vi "Read.vi"(8 "Error In":errorcluster, 10 "Max Data Length":i32=1024, 11 "SFTP File In":refnum<class "SFTP File.lvclass">) -> (0 "Error Out":errorcluster, 2 "Data":u8[](array[numeric]), 3 "SFTP File Out":refnum<class "SFTP File.lvclass">)   [LabVIEW 2021, in "Field_RnD_Services_LIBSSH2_Toolkit.lvlib" / "SFTP File.lvclass"]
doc: "Reads the contents of a remote SFTP file."
uses:
  SFTP File.lvclass
  SFTP File.lvclass/SFTP File.ctl
  Field_RnD_Services_LIBSSH2_Toolkit.lvlib
  SFTP/SFTP.lvclass
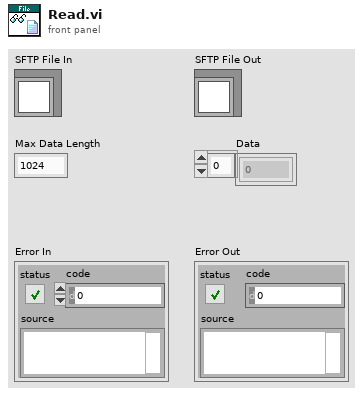
[diagram p1: front panel]
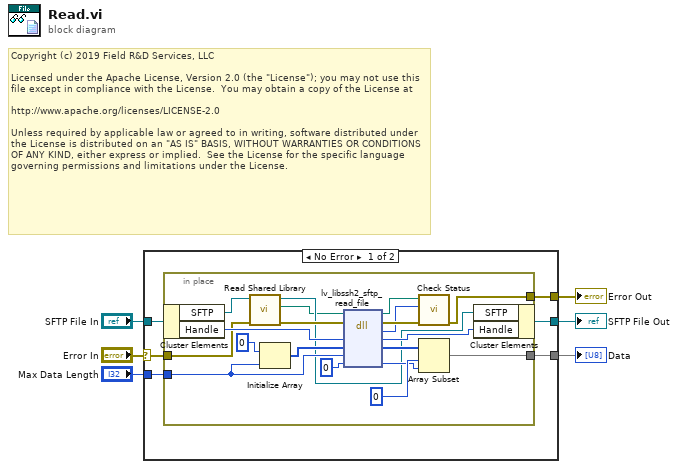
[diagram p0: block diagram]
diagram:
  # "Copyright (c) 2019 Field R&D Services, LLC\n\nLicensed under the Apache License, Version 2.0 (the \"License\"); you may not use this file except in compliance with the License.  You may obtain a copy of the License at\n\nhttp://www.apache.org/licenses/LICENSE-2.0\n\nUnless required by applicable law or agreed to in writing, software distributed under the License is distributed on an \"AS IS\" BASIS, WITHOUT WARRANTIES OR CONDITIONS OF ANY KIND, either express or implied.  See the License for the specific language governing permissions and limitations under the License."
  n1 = case shown="No Error" "Error In" {
    selector: "Error In" -> [w11 w32]
    tunnel: "SFTP File In" -> [w12 w33]
    tunnel: [w10 w33] -> w3
    tunnel: [w7 w32] -> w4
    tunnel: [w9 _] -> w2
    tunnel: "Max Data Length" -> [w8 _]
    frame No Error {
      n2 = in-place {
        in-place-border: w11 -> [w30]
        in-place-border: [w19] -> w9
        in-place-border: w8 -> [w23]
        in-place-border: [w13] -> w7
        n3 = in-place-cluster #1(w12) -> ("SFTP"=w16:refnum<class "SFTP.lvclass">, "Handle"=w31:u64)
        n4 = call "Read Shared Library.vi"("Error In"=w30, "SFTP In"=w16) -> ("Erorr Out"=w17:errorcluster, "libssh2lv Shared Library"=w14:path, "SFTP Out"=w15:refnum<class "SFTP.lvclass">)  [unwired: 7 in]
        n5 = Initialize Array(u8 0, w23) -> (w24:u8[])
        n6 = dll-call lib="D:/Users/cfield/Code/Field R&D Services/SSH/LV-LIBSSH2/LabVIEW/trunk/src/Toolkit/Support/lv-libssh2.*" fn="lv_libssh2_sftp_read_file"(path in=w14, error in=w17, "handle"=w31, "buffer"=w24, "buffer_max_length"=w23, "read_count"=i64 0) -> (path out=w27:path, error out=w28:errorcluster, "status"=w26:i32, "handle"=w29:u64, "buffer"=w21:u8[], "read_count"=w18:i64)  [unwired: 2 in]
        n7 = call "Check Status.vi"("Error In"=w28, "Status"=w26, "libssh2lv Shared Library In"=w27) -> ("Error Out"=w13:errorcluster)  [unwired: 7 in, 1 out]
        n8 = Array Subset(array=w21, index=0, length=w18) -> (w19:u8[])
        n9 = in-place-cluster #1("SFTP"=w15, "Handle"=w29) -> (w10:refnum<class "SFTP File.lvclass">)
      }
    }
    frame Error {
    }
  }
  "Error Out" <- w4
  "SFTP File Out" <- w3
  "Data" <- w2
